vi "AH2500_write_parameters_visa.vi"(4 "error in (no error)":errorcluster caption="Fehler (Eingang, kein Fehler)", 5 "AH2500-Visa-address":refnum<visa-resource-name>, 6 "V excitation":T1(ring), 7 "BIas":enum16{"Disabled", "100 MOhm", "1 MOhm"}(ring), 8 "ALternate":enum16{"0", "1", "2", "3", "4", "5", "6", "7"}(ring)=enum."1", 9 "AVerage":T2(ring)=enum."5") -> (0 "error out":errorcluster caption="Fehler (Ausgang)", 3 "AH2500-Visa-adress-dub":refnum<visa-resource-name>)   [LabVIEW 2018]
uses:
  Global/Global Variables/Data_Display_global.vi
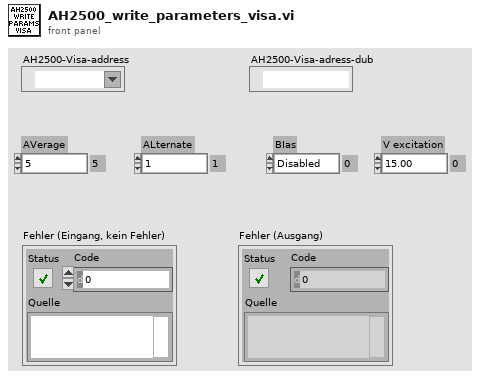
[diagram p1: front panel]
types:
  T1 = enum16{"15.00", "7.50", "3.75", "3.00", "1.50", "0.750", "0.375", "0.250", "0.125", "0.100", "0.050", "0.030", "0.015", "0.010", "0.0050", "0.0030", "0.0015", "0.0010", "0.0005"}
  T2 = enum16{"0", "1", "2", "3", "4", "5", "6", "7", "8", "9", "10", "11", "12", "13", "14", "15"}
  T3 = typedef "AH2500-Cluster.ctl" = cluster{"Capacity Graphic":dbl[][], "Loss Graphic":dbl[][], "Update AH2500":bool, "Capacity":dbl, "Loss":dbl, "AVerage":enum16{"0", "1", "2", "3", "4", "5", "6", "7", "8", "9", "10", "11", "12", "13", "14", "15"}, "ALternate":enum16{"0", "1", "2", "3", "4", "5", "6", "7"}, "BIas":enum16{"Disabled", "100 MOhm", "1 MOhm"}, "V excitation":enum16{"15.00", "7.50", "3.75", "3.00", "1.50", "0.750", "0.375", "0.250", "0.125", "0.100", "0.050", "0.030", "0.015", "0.010", "0.0050", "0.0030", "0.0015", "0.0010", "0.0005"}}
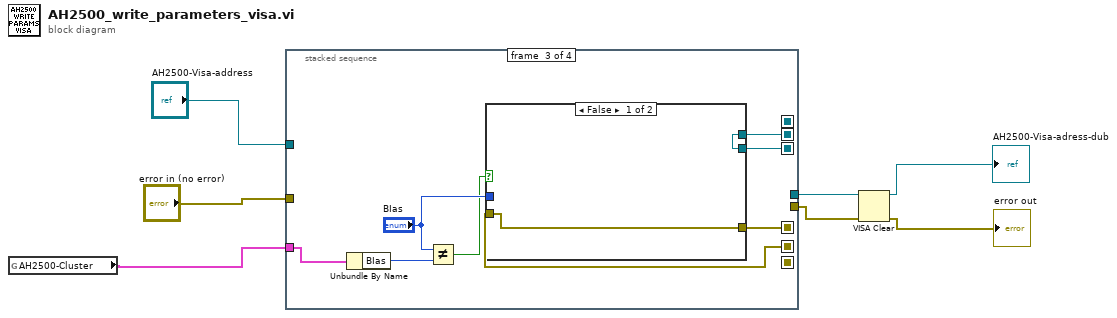
[diagram p0: block diagram]
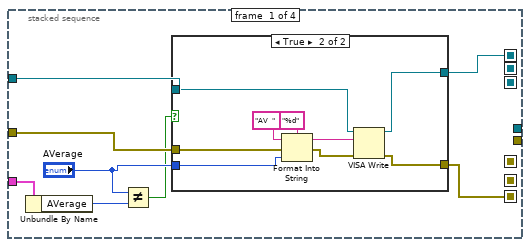
[diagram p2: hidden frame]
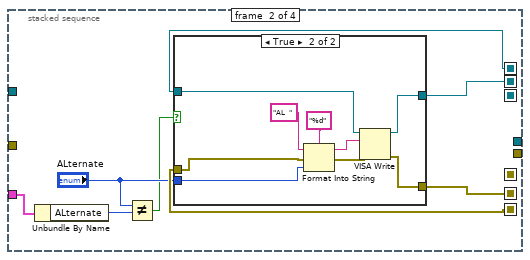
[diagram p4: hidden frame]
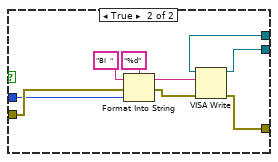
[diagram p6: hidden frame]
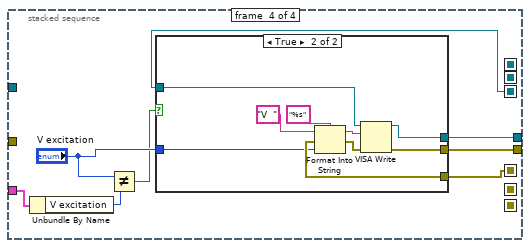
[diagram p7: hidden frame]
diagram:
  n1 = global read "Data_Display_global.vi" "AH2500-Cluster"() -> (w2:T3)
  n2 = stacked-sequence {
    seq-local: [w13 _ _ _] -> [_ w33 _ _]
    seq-local: [w12 _ _ _] -> [_ w34 _ _]
    seq-local: [_ w32 _ _] -> [_ _ w53 _]
    seq-local: [_ w31 _ _] -> [_ _ w46 _]
    seq-local: [_ _ w52 _] -> [_ _ _ w72]
    seq-local: [_ _ w51 _] -> [_ _ _ w71]
    tunnel: "AH2500-Visa-address" -> [w15 _ _ _]
    tunnel: "error in (no error)" -> [w14 _ _ _]
    tunnel: [_ _ _ w70] -> w4
    tunnel: [_ _ _ w69] -> w5
    tunnel: w2 -> [w11 w30 w50 w68]
    frame #0 {
      n3 = Unbundle By Name(w11) -> ("AVerage"=w10:T2)
      n4 = Not Equal?(x="AVerage", y=w10) -> (x != y?=w8:bool)
      n5 = case shown="True" w8 {
        tunnel: w15 -> [w16 w23]
        tunnel: w14 -> [w17 w22]
        tunnel: [w17 w19] -> w13
        tunnel: [w16 w21] -> w12
        tunnel: "AVerage" -> [_ w18]
        frame False {
        }
        frame True {
          n6 = Format Into String(format string="%d", initial string="AV  ", error in=w22, w18) -> (resulting string=w24:string, error out=w20:errorcluster)
          n7 = VISA Write(VISA resource name=w23, write buffer=w24, error in (no error)=w20) -> (VISA resource name out=w21:refnum<visa-resource-name>, error out=w19:errorcluster)  [unwired: 1 out]
        }
      }
    }
    frame #1 {
      n8 = Unbundle By Name(w30) -> ("ALternate"=w28:enum16{"0", "1", "2", "3", "4", "5", "6", "7"})
      n9 = Not Equal?(x="ALternate", y=w28) -> (x != y?=w27:bool)
      n10 = case shown="True" w27 {
        tunnel: w34 -> [w36 w42]
        tunnel: w33 -> [w35 w41]
        tunnel: [w35 w39] -> w32
        tunnel: [w36 w38] -> w31
        tunnel: "ALternate" -> [_ w37]
        frame False {
        }
        frame True {
          n11 = Format Into String(format string="%d", initial string="AL  ", error in=w41, w37) -> (resulting string=w43:string, error out=w40:errorcluster)
          n12 = VISA Write(VISA resource name=w42, write buffer=w43, error in (no error)=w40) -> (VISA resource name out=w38:refnum<visa-resource-name>, error out=w39:errorcluster)  [unwired: 1 out]
        }
      }
    }
    frame #2 {
      n13 = Unbundle By Name(w50) -> ("BIas"=w48:enum16{"Disabled", "100 MOhm", "1 MOhm"})
      n14 = Not Equal?(x="BIas", y=w48) -> (x != y?=w47:bool)
      n15 = case shown="False" w47 {
        tunnel: w53 -> [w55 w61]
        tunnel: [w55 w59] -> w52
        tunnel: [w54 w58] -> w51
        tunnel: "BIas" -> [_ w57]
        tunnel: w46 -> [w54 w56]
        frame False {
        }
        frame True {
          n16 = Format Into String(format string="%d", initial string="BI  ", error in=w61, w57) -> (resulting string=w62:string, error out=w60:errorcluster)
          n17 = VISA Write(VISA resource name=w56, write buffer=w62, error in (no error)=w60) -> (VISA resource name out=w58:refnum<visa-resource-name>, error out=w59:errorcluster)  [unwired: 1 out]
        }
      }
    }
    frame #3 {
      n18 = Unbundle By Name(w68) -> ("V excitation"=w67:T1)
      n19 = Not Equal?(x="V excitation", y=w67) -> (x != y?=w65:bool)
      n20 = case shown="True" w65 {
        tunnel: w71 -> [w73 w80]
        tunnel: w72 -> [w74 w79]
        tunnel: [w74 w77] -> w70
        tunnel: [w73 w76] -> w69
        tunnel: "V excitation" -> [_ w75]
        frame False {
        }
        frame True {
          n21 = Format Into String(format string="%s", initial string="V  ", error in=w79, w75) -> (resulting string=w81:string, error out=w78:errorcluster)
          n22 = VISA Write(VISA resource name=w80, write buffer=w81, error in (no error)=w78) -> (VISA resource name out=w76:refnum<visa-resource-name>, error out=w77:errorcluster)  [unwired: 1 out]
        }
      }
    }
  }
  n23 = VISA Clear(VISA resource name=w5, error in (no error)=w4) -> (VISA resource name out=→"AH2500-Visa-adress-dub":refnum<visa-resource-name>, error out=→"error out":errorcluster)
